vi "RDS Serial Handle Frame.vi"(8 "error in (no error)":errorcluster, 10 "RDS Serial Frame":refnum<class "RDS Serial Frame.lvclass">, 11 "MCB Instrument in":refnum<class "MCB Instrument.lvclass">) -> (0 "error out":errorcluster, 3 "MCB Instrument out":refnum<class "MCB Instrument.lvclass">)   [LabVIEW 2015, in "MCB Instrument.lvlib" / "MCB Instrument.lvclass"]
uses:
  MCB Instrument.lvclass
  Libraries/RDS Serial Handler/RDS Serial Frame.lvclass
  Libraries/RDS Serial Handler/RDS Serial Frame.lvclass/RDS Serial Frame.ctl
  Actors/RDS Parent Actor/RDS Parent Actor/RDS Parent Actor.lvclass
panel:
  out "Serial String":string
  out "x-y":dbl
  out "Time Stamp":timestamp
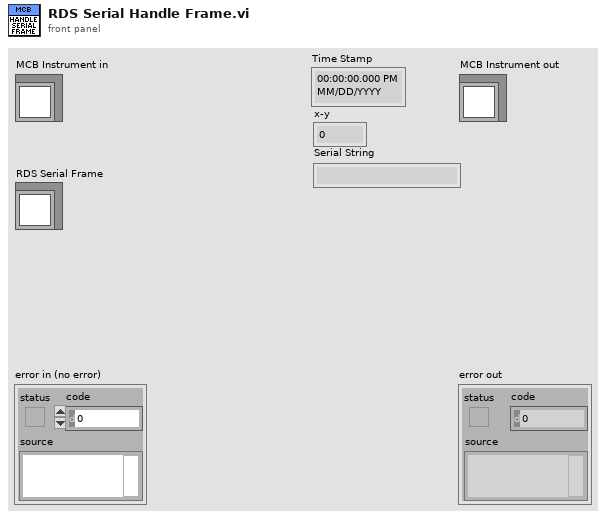
[diagram p1: front panel]
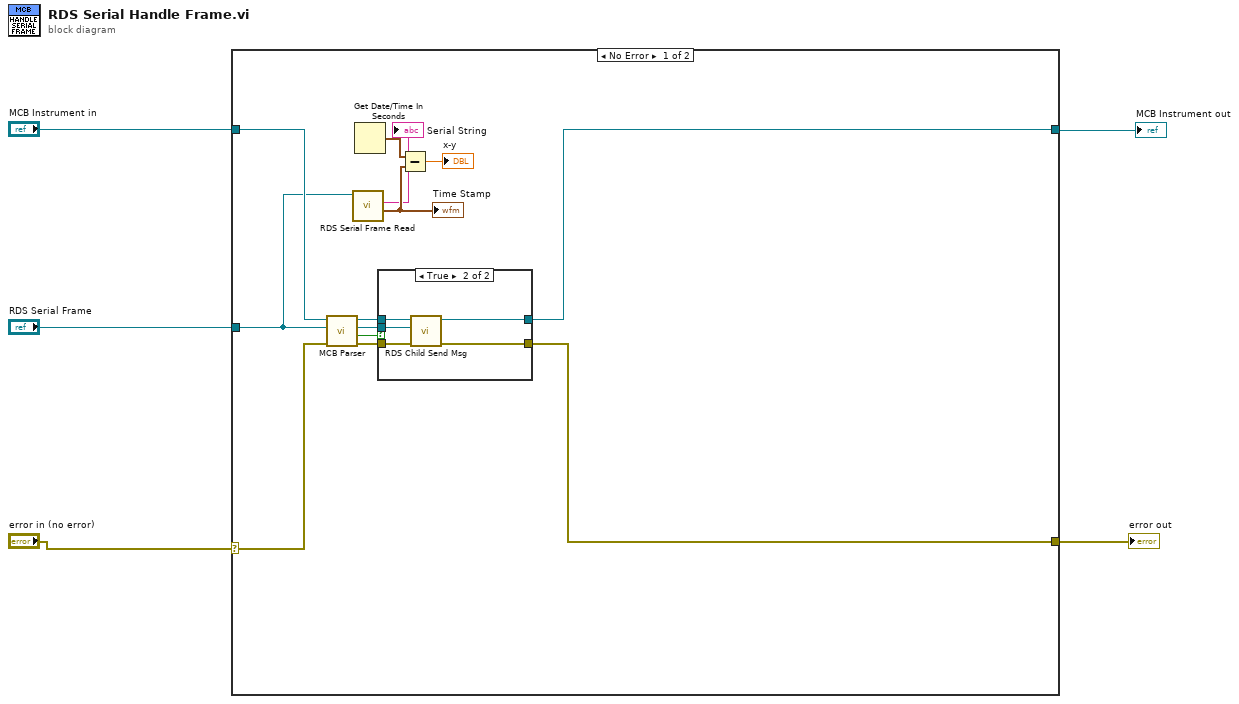
[diagram p0: block diagram]
diagram:
  n1 = case shown="No Error" "error in (no error)" {
    selector: "error in (no error)" -> [w17 w26]
    tunnel: "RDS Serial Frame" -> [w10 _]
    tunnel: "MCB Instrument in" -> [w18 w27]
    tunnel: [w12 w27] -> w2
    tunnel: [w13 w26] -> w1
    frame No Error {
      n2 = call "MCB Parser.vi"("error in (no error)"=w17, "RDS Serial Frame"=w10, "MCB Instrument in"=w18) -> ("error out"=w14:errorcluster, "Valid?"=w11:bool, "RDS Framework.lvlib:RDS Message.lvclass"=w15:refnum<class "RDS Message.lvclass">, "MCB Instrument out"=w16:refnum<class "MCB Instrument.lvclass">)  [unwired: 5 in]
      n3 = call "RDS Serial Frame Read.vi"("RDS Serial Frame in"=w10) -> ("Time Stamp"=w8:timestamp, "Serial String"=→"Serial String":string)  [unwired: 7 in, 2 out]
      "Time Stamp" <- w8
      n4 = Get Date/Time In Seconds() -> (seconds since 1Jan1904=w9:timestamp)
      n5 = case shown="True" w11 {
        tunnel: w16 -> [w20 w25]
        tunnel: w15 -> [_ w24]
        tunnel: w14 -> [w19 w23]
        tunnel: [w19 w22] -> w13
        tunnel: [w20 w21] -> w12
        frame False {
        }
        frame True {
          n6 = call "RDS Child Send Msg.vi"("error in (no error)"=w23, "RDS Message"=w24, "RDS Parent Actor in"=w25) -> ("error out"=w22:errorcluster, "RDS Parent Actor out"=w21:refnum<class "MCB Instrument.lvclass">)  [unwired: 7 in]
        }
      }
      n7 = Subtract(x=w9, y=w8) -> (x-y=→"x-y":dbl)
    }
    frame Error {
    }
  }
  "error out" <- w1
  "MCB Instrument out" <- w2
